vi "Experimental Parameters to XML.vi"() -> (0 "XML Data":string)   [LabVIEW 2013]
uses:
  Types/Experimental Parameters.ctl
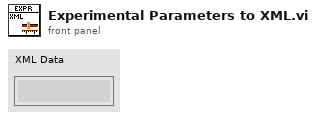
[diagram p1: front panel]
types:
  T1 = typedef "Experimental Parameters.ctl" = cluster{"Number of Samples":dbl, "Ramp Rate":dbl, "Version":string}
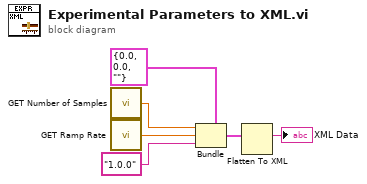
[diagram p0: block diagram]
diagram:
  n1 = call "GET Number of Samples.vi"() -> ("Number of Samples"=w3:dbl)
  n2 = call "GET Ramp Rate.vi"() -> ("Ramp Rate"=w4:dbl)
  n3 = Bundle(cluster=T1 {"Number of Samples"=0.0, "Ramp Rate"=0.0, "Version"=""} ("Experimental Parameters"), "Number of Samples"=w3, "Ramp Rate"=w4, "Version"="1.0.0") -> (w6:T1)
  n4 = Flatten To XML(anything=w6) -> (xml string=→"XML Data":string)
